vi "StringToBoolean.vi"(0 "String":string, 5 "Error In":errorcluster) -> (14 "Boolean":bool, 19 "Error Out":errorcluster)   [LabVIEW 2019]
uses:
  <vilib>/regexp/Match Regular Expression.xnode
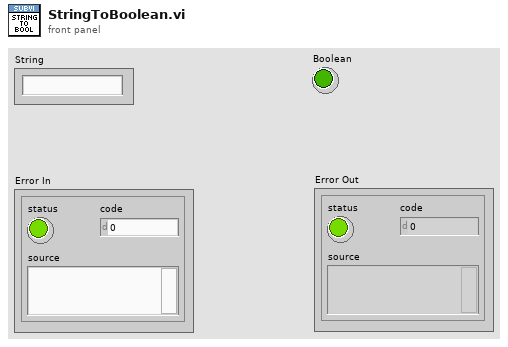
[diagram p1: front panel]
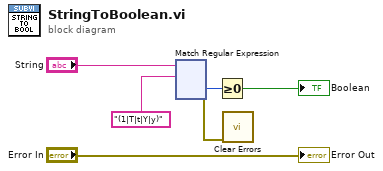
[diagram p0: block diagram]
diagram:
  n1 = xnode "Match Regular Expression"("input string"="String", "regular expression"="(1|T|t|Y|y)") -> ("offset past match"=w5:i32, "error out"=w1:errorcluster)  [unwired: 4 in, 3 out]
  n2 = Greater Or Equal To 0?(x=w5) -> (x >= 0?=→"Boolean":bool)
  n3 = call <vilib>:"Clear Errors.vi"("error in (no error)"=w1) -> ()  [unwired: 5 in, 2 out]
  "Error Out" <- "Error In"
